vi "Utility Write to Instrument.vi"(8 "error in (no error)":errorcluster, 10 "Write Buffer":string, 11 "VISA resource name":refnum<visa-resource-name>) -> (0 "error out":errorcluster, 2 "Read Buffer":string, 3 "VISA resource name out":refnum<visa-resource-name>)   [LabVIEW 2013, in "Berkeley Nucleonics 500 Series.lvlib"]
doc: "This Utility VI is a wrapper which writes to the instrument and reads the response. This VI is intended to be used as a private VI and altering it could cause several public VI's to operate incorrectly."
uses:
  Berkeley Nucleonics 500 Series.lvlib
  <vilib>/Utility/error.llb/DialogType.ctl
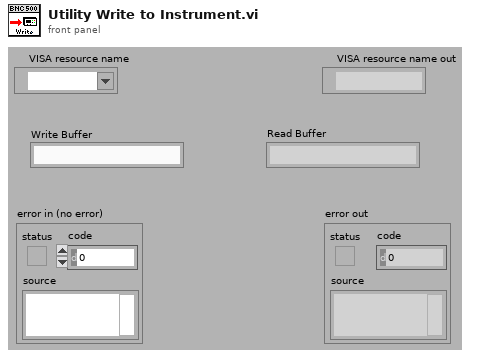
[diagram p1: front panel]
types:
  T1 = typedef "DialogType.ctl" = u16
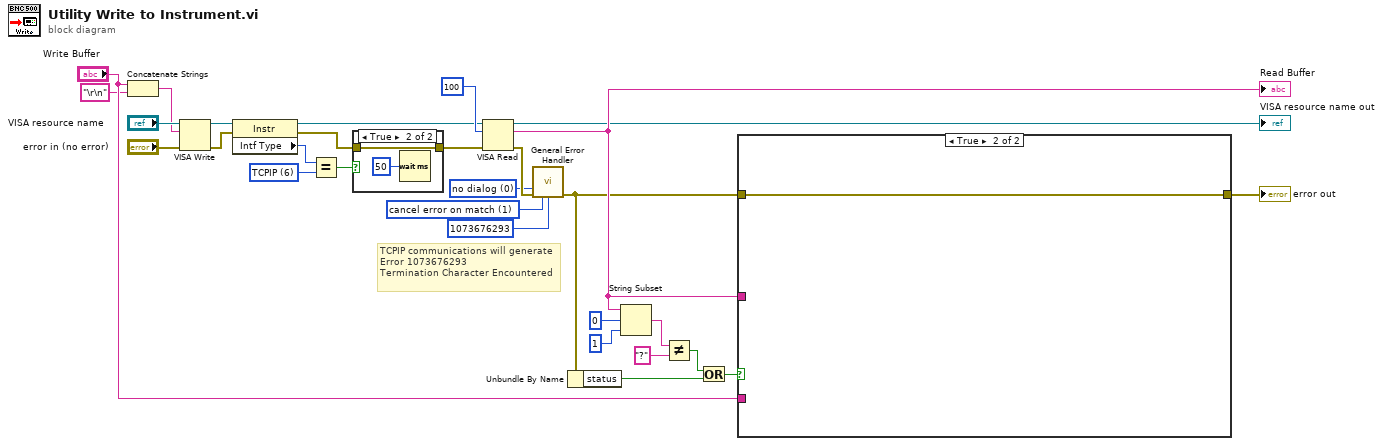
[diagram p0: block diagram]
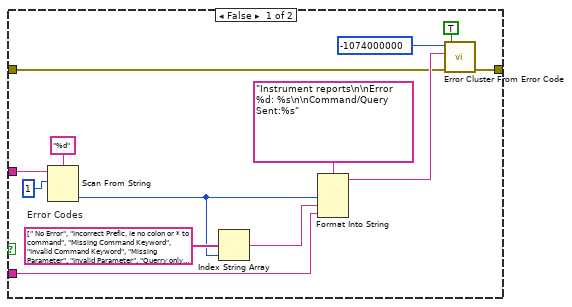
[diagram p3: hidden frame]
diagram:
  w2 = u16 6 items=["GPIB"=1, "VXI"=2, "GPIB-VXI"=3, "Serial"=4, "PXI"=5, "TCPIP"=6, "USB"=7, "FireWire"=9] ("Interface Information:Interface Type")
  w9 = T1 0 items=["no dialog", "OK message", "continue or stop message", "OK message + warnings", "continue/stop + warnings"] ("type of dialog (OK msg:1)")
  w13 = 1 items=["no exception", "cancel error on match", "set error on match"] ("[exception action] (none:0)")
  # "TCPIP communications will generate\nError 1073676293\nTermination Character Encountered"
  n1 = Concatenate Strings("Write Buffer", "\r\n" ("string")) -> (w27:string)
  n2 = VISA Write(VISA resource name="VISA resource name", write buffer=w27, error in (no error)="error in (no error)") -> (VISA resource name out=w6:refnum<visa-resource-name>, error out=w5:errorcluster)  [unwired: 1 out]
  n3 = property class="Instr"(reference=w6, error in=w5) -> (reference out=w4:refnum<visa-resource-name>, error out=w7:errorcluster, "Intf Type"=w1:u16)
  n4 = Equal?(x=w1, y=w2) -> (x = y?=w3:bool)
  n5 = case shown="True" w3 {
    tunnel: [w30 w31] -> w8
    tunnel: w7 -> [w30 w31]
    frame False {
    }
    frame True {
      n6 = Wait (ms)(milliseconds to wait=u32 50) -> ()  [unwired: 1 out]
    }
  }
  n7 = VISA Read(VISA resource name=w4, byte count=u32 100, error in (no error)=w8) -> (VISA resource name out=→"VISA resource name out":refnum<visa-resource-name>, read buffer=w21:string, error out=w10:errorcluster)  [unwired: 1 out]
  "Read Buffer" <- w21
  n8 = call <vilib>:"General Error Handler.vi"("type of dialog (OK msg:1)"=w9, "error in (no error)"=w10, "[exception action] (none:0)"=w13, "[exception code]"=1073676293) -> ("error out"=w11:errorcluster)  [unwired: 7 in, 4 out]
  n9 = Unbundle By Name(w11) -> ("status"=w17:bool)
  n10 = String Subset(string=w21, offset (0)=0, length (rest)=1 ("length (rest)")) -> (substring=w18:string)
  n11 = Not Equal?(x=w18, y="?" ("x")) -> (x != y?=w20:bool)
  n12 = Or(x=w20, y=w17) -> (x .or. y?=w25:bool)
  n13 = case shown="True" w25 {
    tunnel: w21 -> [w44 _]
    tunnel: [w35 w46] -> w24
    tunnel: w11 -> [w33 w46]
    tunnel: "Write Buffer" -> [w39 _]
    frame False {
      w42 = string[] [" No Error", "Incorrect Prefic, ie no colon or * to command", "Missing Command Keyword", "Invalid Command Keyword", "Missing Parameter", "Invalid Parameter", "Querry only, command needs a question mark", "Invalid Query, command does not have a query form"]  # Error Codes
      n14 = Scan From String(format string="%d" ("Format String"), input string=w44, initial scan location=u32 1) -> (output 1=w41:i32)  [unwired: 2 in, 3 out]
      n15 = Index String Array(1:w41, 2:w42) -> (0:w40:string)  [unwired: 1 in]
      n16 = Format Into String(format string="Instrument reports\n\nError %d: %s\n\nCommand/Query Sent:%s" ("Source"), w41, w40, w39) -> (resulting string=w34:string)  [unwired: 2 in, 1 out]
      n17 = call <vilib>:"Error Cluster From Error Code.vi"("show call chain? (False)"=TRUE, "error in (no error)"=w33, "error message (\"\")"=w34, "error code (0)"=-1074000000 ("Code")) -> ("error out"=w35:errorcluster)  [unwired: 5 in]
    }
    frame True {
    }
  }
  "error out" <- w24
